vi "XL320_Save Motion.vi"(8 "Speed Scale":dbl, 9 "Positions":string[][](table), 10 "Step Times":u32[](array[numeric]), 11 "Motor List":u8[](array[numeric])) -> ()   [LabVIEW 2015]
doc: "Saves the positions, motor list, step times, and speed scale of a recorded motion sequence. By default, this VI will save the data as a custom DSQ (Dynamixel Sequence) format. This VI can also export the position data as a tab delimitted text file."
uses:
  <instrlib>/Dynamixel XL320/Examples/Record And Playback Motion/Type Defs/XL320_Raw Motion.ctl
  Instance           1 17Saved   Save File .vi
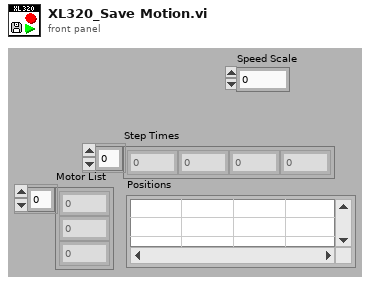
[diagram p1: front panel]
types:
  T1 = typedef "XL320_Raw Motion.ctl" = cluster{"Motor List":u8[], "Gait Positions":string[][], "Gait speeds":u32[], "Speed Scale":dbl}
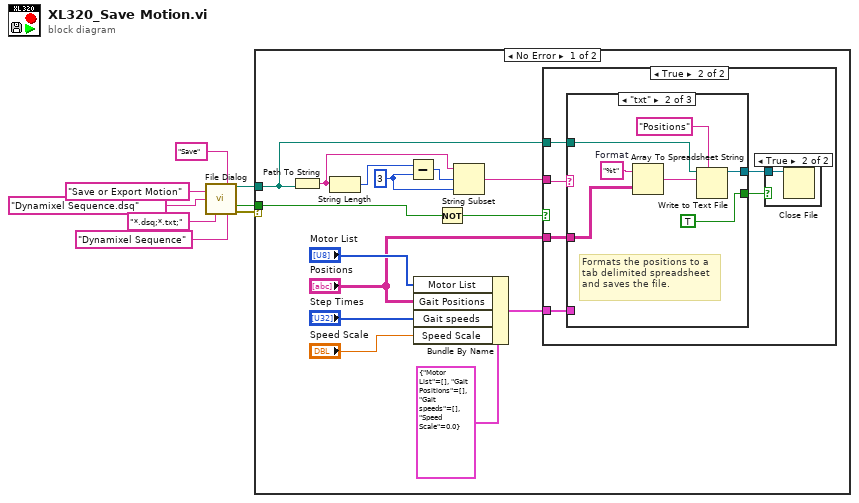
[diagram p0: block diagram]
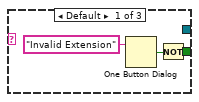
[diagram p4: hidden frame]
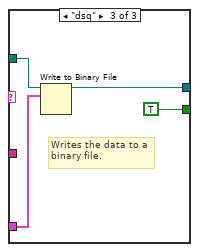
[diagram p5: hidden frame]
diagram:
  n1 = call "File Dialog"("prompt"="Save or Export Motion", "button label"="Save", "default name"="Dynamixel Sequence.dsq", "pattern (all files)"="*.dsq;*.txt;", "pattern label"="Dynamixel Sequence") -> ("selected path"=w5:path, "cancelled"=w7:bool, "error out"=w1:errorcluster)  [unwired: 7 in, 1 out]
  n2 = case shown="No Error" w1 {
    tunnel: w7 -> [w22 _]
    tunnel: w5 -> [w21 _]
    frame No Error {
      w18 = 3 ("length (rest)")
      n3 = Path To String(path=w21) -> (string=w20:string)
      n4 = String Length(string=w20) -> (length=w19:i32)
      n5 = Subtract(x=w19, y=w18) -> (x-y=w17:i32)
      n6 = Bundle By Name(cluster=T1 {"Motor List"=[], "Gait Positions"=[], "Gait speeds"=[], "Speed Scale"=0.0} ("Raw Motion"), "Motor List"="Motor List", "Gait Positions"="Positions", "Gait speeds"="Step Times", "Speed Scale"="Speed Scale") -> (w10:T1)
      n7 = Not(x=w22) -> (.not. x?=w15:bool)
      n8 = String Subset(string=w20, offset (0)=w17, length (rest)=w18) -> (substring=w16:string)
      n9 = case shown="True" w15 {
        tunnel: w21 -> [_ w28]
        tunnel: w16 -> [_ w27]
        tunnel: w10 -> [_ w24]
        tunnel: "Positions" -> [_ w23]
        frame False {
        }
        frame True {
          n10 = case shown="\"txt\"" w27 {
            tunnel: w28 -> [_ w36 w43]
            tunnel: [_ w35 w42] -> w26
            tunnel: [w30 TRUE TRUE] -> w25
            tunnel: w24 -> [_ _ w41]
            tunnel: w23 -> [_ w34 _]
            frame Default {
              n11 = One Button Dialog(message="Invalid Extension") -> (true=w31:bool)  [unwired: 1 in]
              n12 = Not(x=w31) -> (.not. x?=w30:bool)
            }
            frame "txt" {
              w37 = "%t"  # Format
              # "Formats the positions to a\ntab delimited spreadsheet\nand saves the file."
              n13 = Array To Spreadsheet String(array=w34, 3:w37) -> (spreadsheet string=w38:string)  [unwired: 1 in]
              n14 = Write to Text File(prompt (Choose or enter file path)="Positions", file (use dialog)=w36, text=w38) -> (refnum out=w35:refnum<file>)  [unwired: 1 in, 2 out]
            }
            frame "dsq" {
              # "Writes the data to a\nbinary file."
              n15 = Write to Binary File(file (use dialog)=w43, data=w41) -> (refnum out=w42:refnum<file>)  [unwired: 4 in, 2 out]
            }
          }
          n16 = case shown="True" w25 {
            tunnel: w26 -> [_ w29]
            frame False {
            }
            frame True {
              n17 = Close File(refnum=w29) -> ()  [unwired: 1 in, 2 out]
            }
          }
        }
      }
    }
    frame Error {
    }
  }
